vi "Engine - Diesel - Faults Host.vi"() -> ()   [LabVIEW 2015, in "ECS-Host.lvlib"]
uses:
  ECS-Host.lvlib
panel:
  in  "ECT_FaultOverride":bool
  in  "OilP_FaultOverride":bool
  in  "12VPSU_FaultOverride":bool
  in  "BattV_FaultOverride":bool
  in  "5VPSU_FaultOverride":bool
  in  "OilT_FaultOverride":bool
  in  "MAT_FaultOverride":bool
  in  "MAP_FaultOverride":bool
  in  "ExhaustManifoldP_FaultOverride":bool
  in  "EGRDiffP_FaultOverride":bool
  in  "RailP_FaultOverride":bool
  out "TurboSpeed_Warning":bool
  in  "TurboSpeed_MaxNC":sgl caption="Engine Speed" format="%#.3f"
  in  "_TurboSpeed_MinNC":sgl format="%#.3f"
  in  "_TurboSpeed_MinCrit":sgl format="%#.3f"
  out "TurboSpeed":sgl caption="[]" format="%#.3f"
  out "TurboSpeed_CriticalFault":bool
  in  "TurboSpeed_MaxCrit":sgl caption="[]" format="%#.3f"
  out "EGRDiffP_Warning":bool
  in  "EGRDiffP_MaxNC":sgl caption="Oil Pressure" format="%#.3f"
  in  "EGRDiffP_MinNC":sgl format="%#.3f"
  out "EGRDiffP":sgl caption="[]" format="%#.3f"
  out "EGRDiffP_CriticalFault":bool
  in  "EGRDiffP_MinCrit":sgl format="%#.3f"
  in  "EGRDiffP_MaxCrit":sgl caption="[]" format="%#.3f"
  out "EngineSpeed_Warning":bool
  out "OilT_Warning":bool
  out "ECT_Warning":bool
  out "MAT_Warning":bool
  out "MAP_Warning":bool
  out "ExhaustManifoldP_Warning":bool
  out "OilP_Warning":bool
  out "RailP_Warning":bool
  out "5VPSU_Warning":bool
  out "12VPSU_Warning":bool
  out "BattV_Warning":bool
  in  "EngineSpeed_MaxNC":sgl caption="Engine Speed" format="%#.3f"
  in  "ECT_MaxNC":sgl caption="Engine Coolant Temperature" format="%#.3f"
  in  "OilT_MaxNC":sgl caption="Oil Temperature" format="%#.3f"
  in  "MAT_MaxNC":sgl caption="IAT" format="%#.3f"
  in  "MAP_MaxNC":sgl caption="MAP" format="%#.3f"
  in  "ExhaustManifoldP_MaxNC":sgl caption="ExhaustManifoldP" format="%#.3f"
  in  "OilP_MaxNC":sgl caption="Oil Pressure" format="%#.3f"
  in  "RailP_MaxNC":sgl caption="Rail Pressure" format="%#.3f"
  in  "5VPSU_MaxNC":sgl caption="5V Puls BattV" format="%#.3f"
  in  "12VPSU_MaxNC":sgl caption="12V Puls BattV" format="%#.3f"
  in  "BattV_MaxNC":sgl caption="TDK BattV" format="%#.3f"
  in  "_EngineSpeed_MinNC":sgl format="%#.3f"
  in  "ECT_MinNC":sgl format="%#.3f"
  in  "OilT_MinNC":sgl format="%#.3f"
  in  "MAT_MinNC":sgl format="%#.3f"
  in  "MAP_MinNC":sgl format="%#.3f"
  in  "ExhaustManifoldP_MinNC":sgl format="%#.3f"
  in  "OilP_MinNC":sgl format="%#.3f"
  in  "RailP_MinNC":sgl format="%#.3f"
  in  "5VPSU_MinNC":sgl format="%#.3f"
  in  "12VPSU_MinNC":sgl format="%#.3f"
  in  "BattV_MinNC":sgl format="%#.3f"
  in  "_EngineSpeed_MinCrit":sgl format="%#.3f"
  out "EngineSpeed":sgl caption="[]" format="%#.3f"
  out "ECT":sgl caption="[]" format="%#.3f"
  out "OilT":sgl caption="[]" format="%#.3f"
  out "MAT":sgl caption="[]" format="%#.3f"
  out "MAP":sgl caption="[]" format="%#.3f"
  out "ExhaustManifoldP":sgl caption="[]" format="%#.3f"
  out "OilP":sgl caption="[]" format="%#.3f"
  out "RailP":sgl caption="[]" format="%#.3f"
  out "5VPSU":sgl caption="[]" format="%#.3f"
  out "12VPSU":sgl caption="[]" format="%#.3f"
  out "BattV":sgl caption="[]" format="%#.3f"
  out "EngineSpeed_CriticalFault":bool
  out "OilT_CriticalFault":bool
  out "ECT_CriticalFault":bool
  out "MAT_CriticalFault":bool
  out "MAP_CriticalFault":bool
  out "ExhaustManifoldP_CriticalFault":bool
  out "OilP_CriticalFault":bool
  out "RailP_CriticalFault":bool
  out "5VPSU_CriticalFault":bool
  out "12VPSU_CriticalFault":bool
  out "BattV_CriticalFault":bool
  in  "EngineSpeed_MaxCrit":sgl caption="[]" format="%#.3f"
  in  "ECT_MinCrit":sgl format="%#.3f"
  in  "OilT_MinCrit":sgl format="%#.3f"
  in  "ECT_MaxCrit":sgl caption="[]" format="%#.3f"
  in  "OilT_MaxCrit":sgl caption="[]" format="%#.3f"
  in  "MAT_MinCrit":sgl format="%#.3f"
  in  "MAP_MinCrit":sgl format="%#.3f"
  in  "ExhaustManifoldP_MinCrit":sgl format="%#.3f"
  in  "OilP_MinCrit":sgl format="%#.3f"
  in  "MAT_MaxCrit":sgl caption="[]" format="%#.3f"
  in  "MAP_MaxCrit":sgl caption="[]" format="%#.3f"
  in  "ExhaustManifoldP_MaxCrit":sgl caption="[]" format="%#.3f"
  in  "OilP_MaxCrit":sgl caption="[]" format="%#.3f"
  in  "RailP_MinCrit":sgl format="%#.3f"
  in  "5VPSU_MinCrit":sgl format="%#.3f"
  in  "12VPSU_MinCrit":sgl format="%#.3f"
  in  "BattV_MinCrit":sgl format="%#.3f"
  in  "RailP_MaxCrit":sgl caption="[]" format="%#.3f"
  in  "5VPSU_MaxCrit":sgl caption="[]" format="%#.3f"
  in  "12VPSU_MaxCrit":sgl caption="[]" format="%#.3f"
  in  "BattV_MaxCrit":sgl caption="[]" format="%#.3f"
  # "Critical\nMin"
  # "Non-Crit\nMin"
  # "Actual \nValue"
  # "Non-Crit\nMax"
  # "Critical\nMax"
  # "Non-Crit\nWarning"
  # "Critical\nFault"
  # "BattV"
  # "12V PSU"
  # "5V PSU"
  # "Rail Pressure"
  # "Oil Pressure"
  # "EGR Differential Pressure"
  # "Exhaust Manifold Pressure"
  # "MAP"
  # "MAT"
  # "Oil Temperature"
  # "Engine Coolant Temperature"
  # "Engine Speed"
  # "Turbocharger Speed"
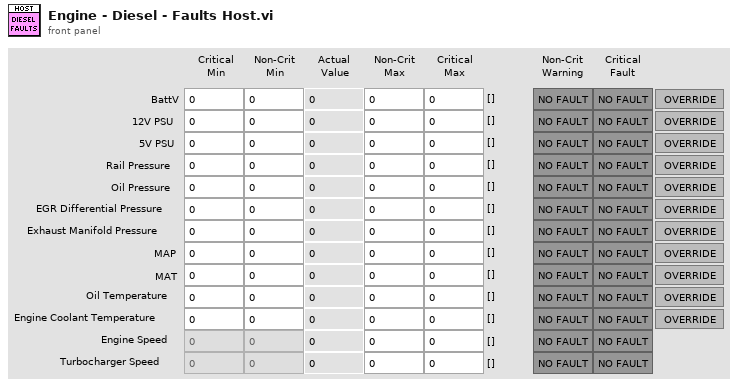
[diagram p1: front panel]
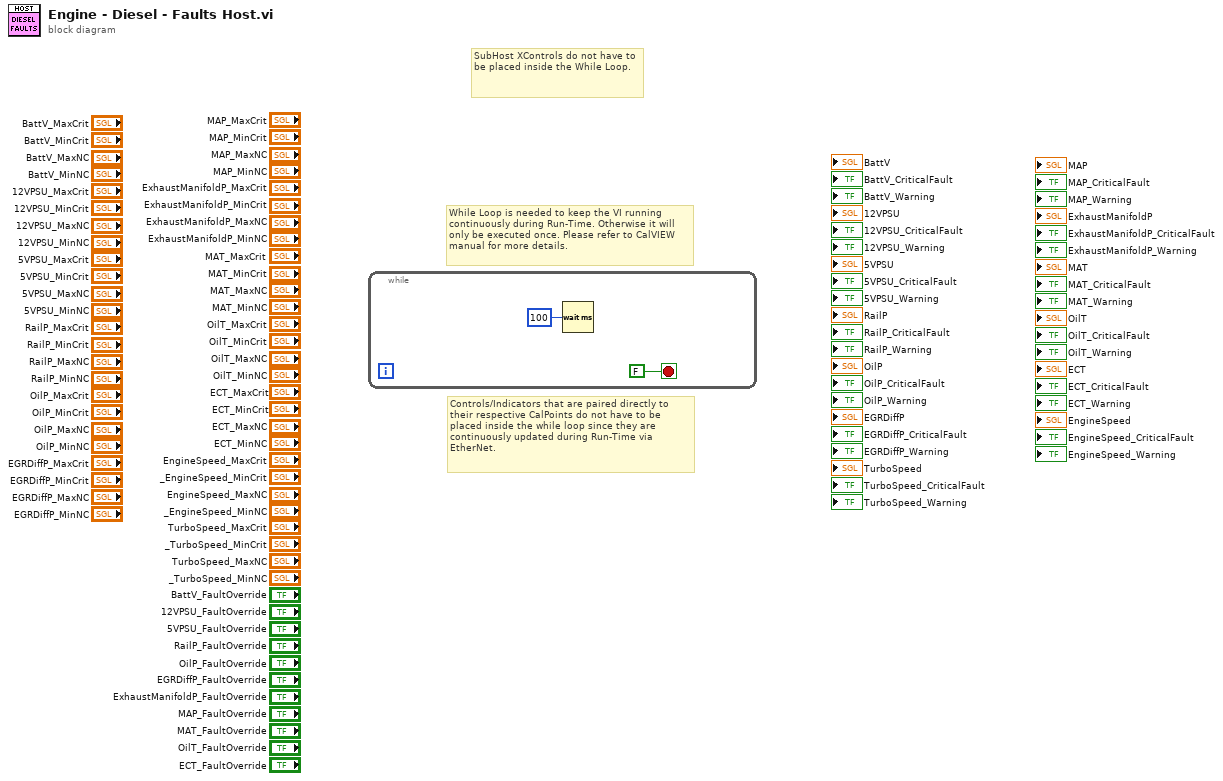
[diagram p0: block diagram]
diagram:
  # "Controls/Indicators that are paired directly to their respective CalPoints do not have to be placed inside the while loop since they are continuously updated during Run-Time via EtherNet."
  # "SubHost XControls do not have to be placed inside the While Loop."
  # "While Loop is needed to keep the VI running\ncontinuously during Run-Time. Otherwise it will only be executed once. Please refer to CalVIEW manual for more details."
  n1 = while {
    stop <- FALSE stop-if-true
    n2 = Wait (ms)(milliseconds to wait=u32 100 ("millisecond timer value")) -> ()  [unwired: 1 out]
  }
